vi "Init System.vi"(8 "error in (no error)":errorcluster, 11 "System SAL in":refnum<class "System SAL.lvclass">) -> (0 "error out":errorcluster, 3 "System SAL out":refnum<class "System SAL.lvclass">)   [LabVIEW 2020, in "Volatus.lvlib" / "System SAL.lvclass"]
uses:
  System SAL.lvclass
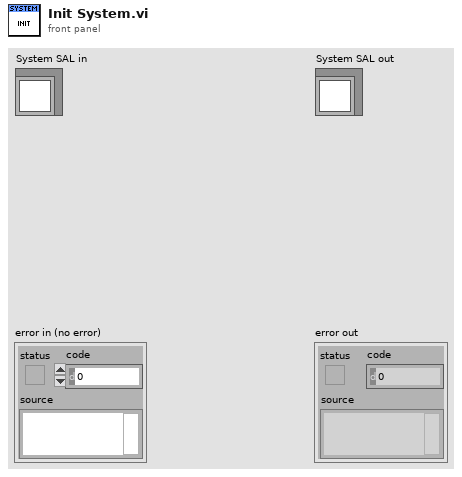
[diagram p1: front panel]
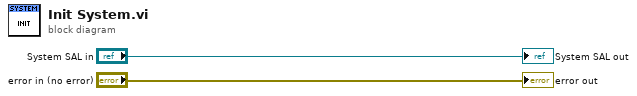
[diagram p0: block diagram]
diagram:
  "error out" <- "error in (no error)"
  "System SAL out" <- "System SAL in"
